vi "Pirani Gauge Reader.vi"(11 "Trigger Pressure":dbl=2.0) -> (1 "Filament Fault":bool, 2 "Pressure  (Torr)":dbl=0.19 format="%#_6e", 3 "Trigger":bool)   [LabVIEW 2011]
uses:
  <vilib>/Utility/file.llb/Read From Spreadsheet File (DBL).vi
  <vilib>/imath/engines/lvmath2/RunTimeEngine/ErrorHandling/NIMS_Finalize Error.vi
  <vilib>/imath/engines/lvmath2/RunTimeEngine/Managers/WorkSpace/UID Generator.vi
  <vilib>/imath/engines/lvmath2/RunTimeEngine/Managers/SymbolTable/Clear UID.vi
  <vilib>/imath/engines/lvmath2/RunTimeEngine/NodeEndStatement/NIMS_NodeEndStatement_Output.vi
  <instcachedir>/0/NIMS_NodeEndStatement_Output_53EC0D466D134D7ABD903AC30B43404B.lvgen/NIMS_NodeEndStatement_Output_53EC0D466D134D7ABD903AC30B43404B_001.vi
  <vilib>/imath/engines/lvmath2/RunTimeEngine/VariableToken/Read/NIMS_Get Elements - RV(_) - Check(_).vi
  <instcachedir>/0/NIMS_Get Elements - RV(_) - Check(_)_95E78A4FFA0646428F3543E57837F638.lvgen/NIMS_Get Elements - RV(_) - Check(_)_95E78A4FFA0646428F3543E57837F638_000.vi
  <vilib>/imath/engines/lvmath2/RunTimeEngine/RunTimeType/NIMS_RunTimeType_From StrictType (excl LVString).vi
  <instcachedir>/0/NIMS_RunTimeType_From StrictType (excl LVString)_46AE8B54A11948F0BCCEB8091EE7AA4C.lvgen/NIMS_RunTimeType_From StrictType (excl LVString)_46AE8B54A11948F0BCCEB8091EE7AA4C_000.vi
  <vilib>/imathl/engines/lvmath/Functions/Error Handling/Create Error.vi
  <vilib>/imath/engines/lvmath2/RunTimeEngine/LocalVariableDefStatement/MC_LocalVariableDefStatement_Display.vi
  <vilib>/imath/engines/lvmath2/RunTimeEngine/Managers/SymbolTable/NIMS_WorkSpace.lvlib
panel:
  out "?":dbl(graph)
  out "Trig Red":bool
  out "Pressure  (Torr)":dbl(knob)=760.0 scale=0.001..760.0 scale format="%#_6e"
  in  "stop":bool
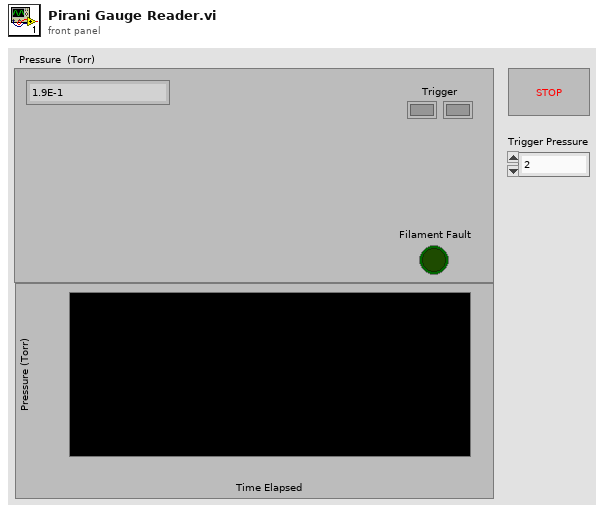
[diagram p1: front panel]
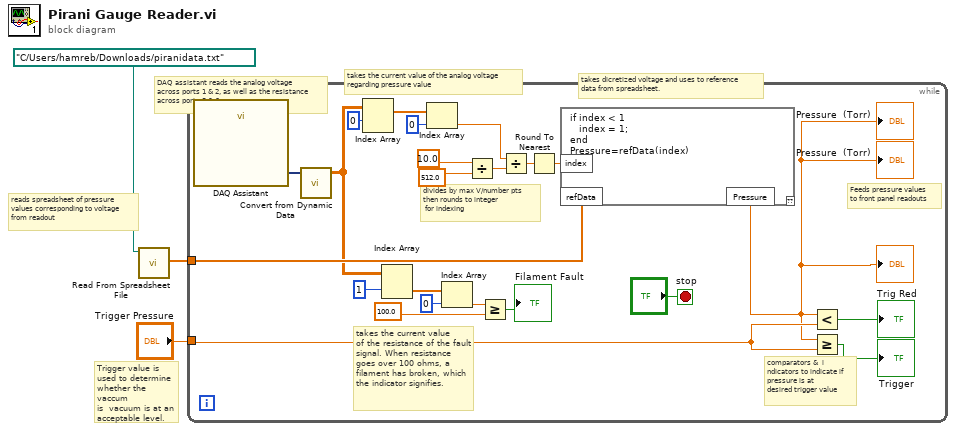
[diagram p0: block diagram]
diagram:
  # "Trigger value is\nused to determine\nwhether the vaccum\nis  vacuum is at an\nacceptable level."
  # "takes dicretized voltage and uses to reference \ndata from spreadsheet."
  # "reads spreadsheet of pressure\nvalues corresponding to voltage \nfrom readout"
  # "DAQ assistant reads the analog voltage \nacross ports 1 & 2, as well as the resistance\nacross ports 5 & 6"
  # "takes the current value of the analog voltage\nregarding pressure value"
  n1 = call-poly <vilib>:"Read From Spreadsheet File.vi"("file path (dialog if empty)"=path "C:/Users/hamreb/Downloads/piranidata.txt") -> ("first row"=w2:dbl[])  [unwired: 6 in, 4 out]
  n2 = while {
    tunnel: w2 -> [w25]
    tunnel: "Trigger Pressure" -> [w19]
    stop <- "stop" stop-if-true
    # "divides by max V/number pts \nthen rounds to integer\n for indexing"
    # "Feeds pressure values\nto front panel readouts"
    # "takes the current value \nof the resistance of the fault\nsignal. When resistance goes over 100 ohms, a filament has broken, which the indicator signifies."
    # "comparators &  i\nndicators to indicate if \npressure is at\ndesired trigger value"
    n3 = call "DAQ Assistant"() -> ("data"=w17:dynamicdata)  [unwired: 16 in, 3 out]
    n4 = call "Convert from Dynamic Data"("Dynamic Data Type"=w17) -> ("Array"=w16:dbl[][])  [unwired: 3 in]
    n5 = Index Array(array=w16, index (row)=0) -> (element=w13:dbl[])  [unwired: 1 in]
    n6 = Index Array(array=w16, index (row)=1) -> (element=w10:dbl[])  [unwired: 1 in]
    n7 = Index Array(array=w13, index=0) -> (element=w11:dbl)
    n8 = Index Array(array=w10, index=0) -> (element=w8:dbl)
    n9 = Divide(x=10.0, y=512.0) -> (x/y=w23:dbl)
    n10 = Greater Or Equal?(x=w8, y=100.0) -> (x >= y?=→"Filament Fault":bool)
    n11 = Divide(x=w11, y=w23) -> (x/y=w22:dbl)
    n12 = Round To Nearest(number=w22) -> (nearest integer value=w21:dbl)
    n13 = mathscript code="if index < 1\n   index = 1;\nend\nPressure=refData(index)"("refData"=w25, "index"=w21) -> ("Pressure"=w4:dbl)  [unwired: 1 in, 1 out]
    "Pressure  (Torr)" <- w4
    "Pressure  (Torr)" <- w4
    "?" <- w4
    n14 = Less?(x=w4, y=w19) -> (x < y?=→"Trig Red":bool)
    n15 = Greater Or Equal?(x=w4, y=w19) -> (x >= y?=→"Trigger":bool)
  }
